vi "Read Gyro X.vi"() -> ()   [LabVIEW 2015]
uses:
  <vilib>/myRIO/Instrument Drivers/Onboard IO/I2C/typedefs/I2C User Configuration.ctl
  <vilib>/myRIO/Instrument Drivers/Onboard IO/I2C/typedefs/I2C Transfer Rate.ctl
  <vilib>/myRIO/Instrument Drivers/Onboard IO/I2C/typedefs/I2C Reference.ctl
  <vilib>/myRIO/Common/Instrument Driver Framework/Utilities/typedefs/myRIO Generic Hardware Reference.ctl
  <vilib>/myRIO/Common/Instrument Driver Framework/Utilities/typedefs/Hardware Version Enum.ctl
  <vilib>/myRIO/Common/Instrument Driver Framework/Utilities/typedefs/myRIO v1.0 Reference.ctl
  <vilib>/myRIO/Common/Instrument Driver Framework/Utilities/typedefs/Generic FPGA Reference.ctl
  <vilib>/myRIO/Common/Instrument Driver Framework/myRIO v1.0/I2C/typedefs/I2C Channels Enum.ctl
  <vilib>/myRIO/Instrument Drivers/Onboard IO/I2C/typedefs/I2C Configuration.ctl
  <vilib>/userdefined/High Color/nirio_resource_hc.ctl
  <vilib>/Platform/TimedLoop/XDataNode/timing_clust.ctl
  <vilib>/Platform/TimedLoop/XDataNode/nitl_modes.ctl
  <vilib>/Platform/TimedLoop/XDataNode/wakeup.ctl
  <vilib>/myRIO/Common/Instrument Driver Framework/myRIO v1.0/I2C/vis/myRIO v1.1 Open I2C.vi
  <vilib>/myRIO/Common/Instrument Driver Framework/Utilities/vis/Validate Channels.vi
  <vilib>/myRIO/Common/Instrument Driver Framework/myRIO v1.0/I2C/vis/myRIO v1.0 Reserve I2C.vi
  <vilib>/myRIO/Common/Instrument Driver Framework/myRIO v1.0/I2C/vis/myRIO v1.0 Build MUX Configuration I2C.vi
  <vilib>/myRIO/Common/Instrument Driver Framework/myRIO v1.0/Resource Manager/vis/myRIO v1.0 Reserve Channel List.vi
  <vilib>/myRIO/Common/Instrument Driver Framework/myRIO v1.0/Resource Manager/vis/myRIO v1.0 Create Configuration List.vi
  <vilib>/myRIO/Common/Instrument Driver Framework/myRIO v1.0/Resource Manager/vis/myRIO v1.0 Reserve Channel.vi
  <vilib>/myRIO/Common/Instrument Driver Framework/myRIO v1.0/Resource Manager/vis/myRIO v1.0 Unreserve Channel.vi
  <vilib>/myRIO/Common/Instrument Driver Framework/myRIO v1.0/Resource Manager/vis/myRIO v1.0 Build Mutex Name.vi
  <vilib>/Utility/VariantDataType/GetNumericInfo.vi
  <vilib>/Utility/error.llb/Error Cluster From Error Code.vi
  <vilib>/myRIO/Common/Instrument Driver Framework/myRIO v1.0/myRIO v1.1 Open.vi
  <vilib>/myRIO/Common/Instrument Driver Framework/Utilities/vis/IO Manager.vi
  <vilib>/myRIO/Common/Instrument Driver Framework/Utilities/vis/Configuration Manager.vi
  <vilib>/myRIO/Common/Instrument Driver Framework/myRIO v1.0/Resource Manager/vis/myRIO v1.0 Configure IO.vi
  <vilib>/myRIO/Common/Instrument Driver Framework/myRIO v1.0/myRIO v1.0 Close.vi
  <vilib>/myRIO/Common/Instrument Driver Framework/myRIO v1.0/I2C/vis/myRIO v1.0 Configure I2C.vi
  <vilib>/myRIO/Common/Instrument Driver Framework/myRIO v1.0/I2C/vis/myRIO v1.0 Write I2C.vi
  <vilib>/myRIO/Common/Instrument Driver Framework/myRIO v1.0/I2C/vis/myRIO v1.0 Read I2C.vi
  <vilib>/myRIO/Instrument Drivers/Onboard IO/I2C/vis/myRIO I2C Open.xnode
  <vilib>/platform/TimedLoop/XDataNode/XDataNode.xnode
  <vilib>/myRIO/Instrument Drivers/Onboard IO/I2C/I2C.lvlib
  <vilib>/Platform/TimedLoop/XDataNode/XDNodeRunTimeDep.lvlib
panel:
  out "atan2 y, x - adjusted":dbl
  out "z":i16
  out "x":i16
  out "y":i16
  out "Numeric":i32
  in  "stop":bool
  out "Bytes Read":u8[](array[numeric]) format="%b"
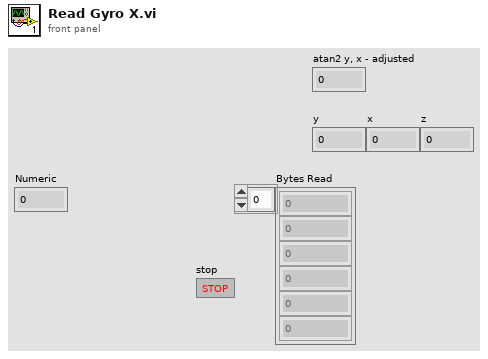
[diagram p1: front panel]
types:
  T1 = typedef "I2C.lvlib/I2C User Configuration.ctl" = cluster{"I2C Transfer Rate":T2}
  T2 = typedef "I2C.lvlib/I2C Transfer Rate.ctl" = enum16{"Standard mode (100 kbps)", "Fast mode (400 kbps)"}
  T3 = typedef "nirio_resource_hc.ctl" = tag
  T4 = typedef "Hardware Version Enum.ctl" = enum16{"Unknown", "myRIO-1900", "myRIO-1950", "roboRIO"}
  T5 = typedef "XDNodeRunTimeDep.lvlib/timing_clust.ctl" = cluster{"Expected End [f-1]":u64, "Actual End [f-1]":u64, "Finished Late? [f-1]":bool, "Expected End [i-1]":u64, "Actual End [i-1]":u64, "Finished Late? [i-1]":bool, "Expected Start [i]":u64, "Actual Start [i]":u64, "Expected Start [f]":u64, "Actual Start [f]":u64, "Source Name":string, "Structure Name":string, "Period":i64, "Deadline":i64, "Offset":i64, "Start":i64, "Priority":i32, "Timeout":i32, "Mode":T6, "Wakeup Reason":T7, "Error":errorcluster, "Source Type":string, "Secondary Source Type":string, "Global End Time":u64, "Global Start Time":u64, "Frame Duration":u64, "Iteration Duration":u64, "Assigned CPU":i32, "I/O Scan Engine Mode":u32}
  T6 = typedef "XDNodeRunTimeDep.lvlib/nitl_modes.ctl" = enum32{"No Change", "Process missed periods, maintain original phase", "Discard missed periods, maintain original phase", "Process missed periods, ignore original phase", "Discard missed periods, ignore original phase"}
  T7 = typedef "XDNodeRunTimeDep.lvlib/wakeup.ctl" = enum32{"Normal", "Aborted", "Asynchronous wakeup", "Timing source error", "Timed loop error", "Timeout"}
  T8 = typedef "I2C.lvlib/I2C Reference.ctl" = cluster{"myRIO Reference":T9, "I2C Channels Enum":T12, "I2C Configuration":T13}
  T9 = typedef "myRIO Generic Hardware Reference.ctl" = cluster{"myRIO Model":T4, "myRIO Hardware Reference":T10}
  T10 = typedef "myRIO v1.0 Reference.ctl" = cluster{"Generic FPGA Reference":T11, "Allow multiple opens":bool}
  T11 = typedef "Generic FPGA Reference.ctl" = refnum<k20>
  T12 = typedef "I2C Channels Enum.ctl" = enum16{"Not Connected", "A/I2C", "B/I2C", "I2C/I2C"}
  T13 = typedef "I2C.lvlib/I2C Configuration.ctl" = cluster{"I2C Transfer Rate":T2}
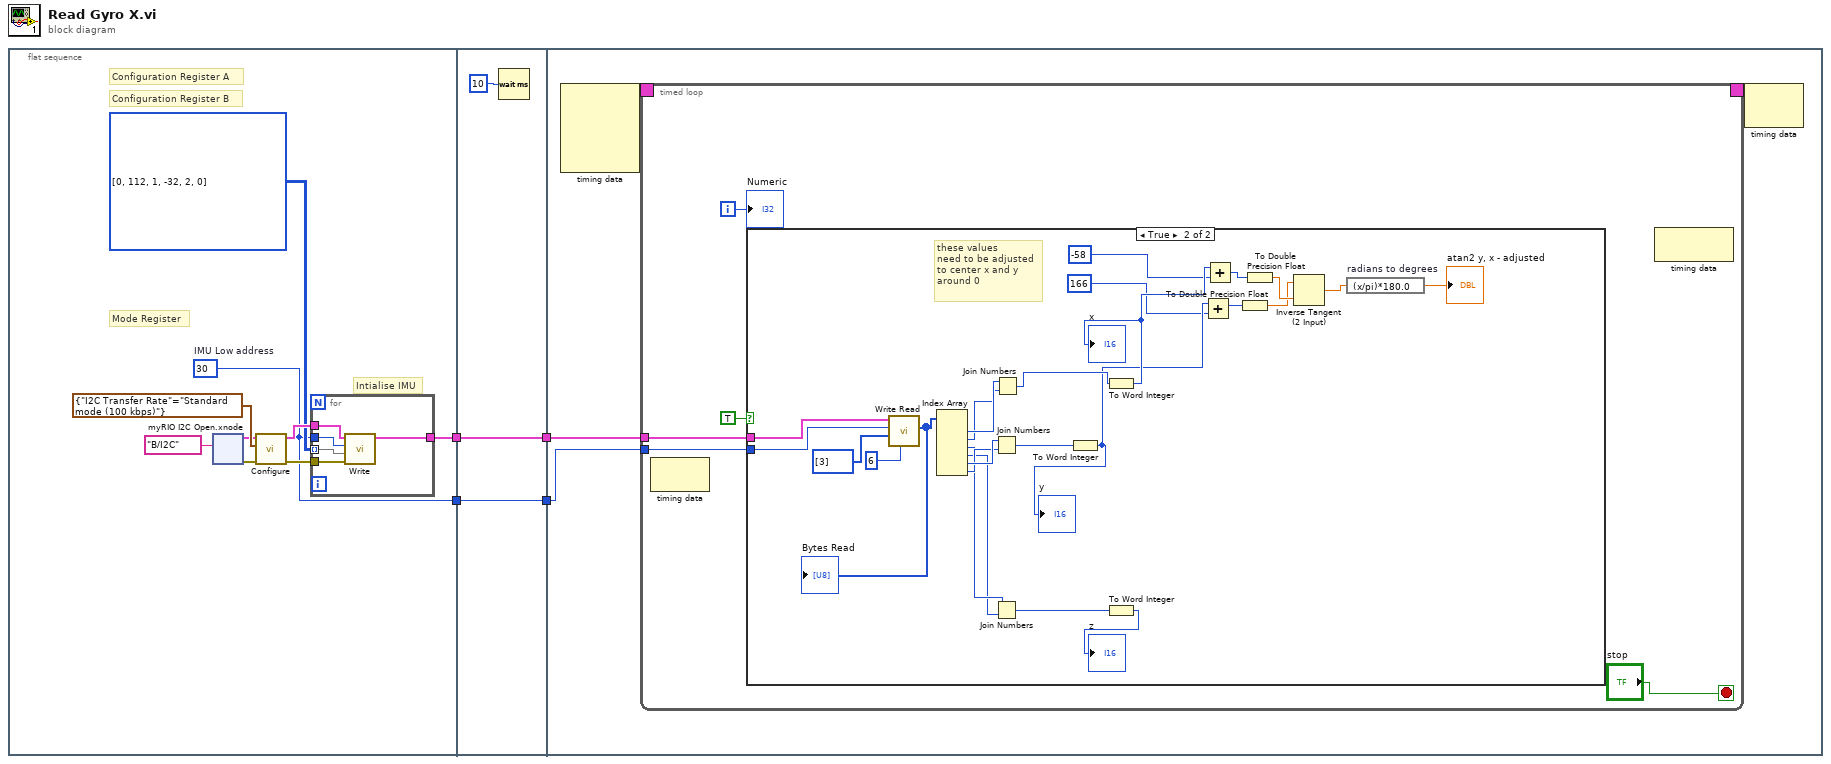
[diagram p0: block diagram]
diagram:
  n1 = flat-sequence {
    tunnel: [w6] -> w4
    tunnel: [w5] -> w2
    tunnel: w4 -> [w37]
    tunnel: [w37] -> w3
    tunnel: w2 -> [w36]
    tunnel: [w36] -> w1
    tunnel: w3 -> [w39]
    tunnel: w1 -> [w38]
    frame #0 {
      w5 = u8 30  # IMU Low address
      # "Mode Register"
      # "Intialise IMU"
      # "Configuration Register B"
      # "Configuration Register A"
      n2 = xnode "myRIO I2C Open.xnode"("Channel Name"=tag "B/I2C") -> ("error out"=w12:errorcluster, "I2C Ref Out"=w8:T8)  [unwired: 2 in]
      n3 = call <vilib>:"Configure.vi"("error in (no error)"=w12, "I2C User Configuration"=T1 {"I2C Transfer Rate"=enum."Standard mode (100 kbps)"}, "I2C Ref In"=w8) -> ("error out"=w13:errorcluster, "I2C Ref Out"=w11:T8)  [unwired: 7 in]
      n4 = for {
        tunnel: i8[][] [[0, 112], [1, -32], [2, 0]] -> [w18] mode=indexing
        tunnel: w11 -> [w17]
        tunnel: w5 -> [w16]
        tunnel: w13 -> [w15]
        tunnel: [w14] -> w6
        n5 = call <vilib>:"Write.vi"("error in (no error)"=w15, "Bytes to Write"=w18, "Slave Address (7-bit)"=w16, "I2C Ref In"=w17) -> ("I2C Ref Out"=w14:T8)  [unwired: 6 in, 1 out]
      }
    }
    frame #1 {
      n6 = Wait (ms)(milliseconds to wait=u32 10) -> ()  [unwired: 1 out]
    }
    frame #2 {
      n7 = node-c288() -> (w41:T5)  [unwired: 4 in]
      n8 = timed-loop {
        timing: w41 -> [_]
        timing-out: [_] -> w40
        tunnel: w39 -> [w46]
        tunnel: w38 -> [w45]
        i -> [w43]
        stop <- "stop" stop-if-true
        n9 = node-c288() -> ()  [unwired: 1 in, 1 out]
        n10 = case shown="True" TRUE {
          tunnel: w46 -> [_ w71]
          tunnel: w45 -> [_ w70]
          frame False {
          }
          frame True {
            # "these values\nneed to be adjusted\nto center x and y\naround 0"
            n11 = call <vilib>:"Write Read.vi"("Byte Count"=u32 6, "Bytes to Write"=u8[] [3], "Slave Address (7-bit)"=w70, "I2C Ref In"=w71) -> ("Bytes Read"=w62:u8[])  [unwired: 4 in, 2 out]
            "Bytes Read" <- w62
            n12 = Index Array(array=w62) -> (element #1=w65:u8, element #2=w64:u8, element #3=w59:u8, element #4=w58:u8, element #5=w61:u8, element #6=w60:u8)  [unwired: 6 in]
            n13 = Join Numbers(hi=w61, lo=w60) -> ((hi.lo)=w67:u16)
            n14 = Join Numbers(hi=w59, lo=w58) -> ((hi.lo)=w66:u16)
            n15 = Join Numbers(hi=w65, lo=w64) -> ((hi.lo)=w63:u16)
            n16 = To Word Integer(number=w67) -> (16bit integer=w55:i16)
            "y" <- w55
            n17 = To Word Integer(number=w63) -> (16bit integer=w56:i16)
            "x" <- w56
            n18 = To Word Integer(number=w66) -> (16bit integer=→"z":i16)
            n19 = Add(x=w55, y=i16 166) -> (x+y=w50:i16)
            n20 = Add(x=w56, y=i16 -58) -> (x+y=w52:i16)
            n21 = To Double Precision Float(number=w50) -> (double precision float=w49:dbl)
            n22 = To Double Precision Float(number=w52) -> (double precision float=w51:dbl)
            n23 = Inverse Tangent (2 Input)(1:w51, 2:w49) -> (0:w48:dbl)
            n24 = expression code="(x/pi)*180.0" "radians to degrees"(w48) -> (→"atan2 y, x - adjusted":dbl)
          }
        }
        n25 = node-c288() -> ()  [unwired: 1 in, 1 out]
        "Numeric" <- w43
      }
      n26 = node-c288(w40) -> ()  [unwired: 1 out]
    }
  }
